vi "medicao.vi"() -> ()   [LabVIEW 2023]
doc: "This example performs writes and reads on a serial port, as directed by the user. You can press the Write and Read buttons, and change the Read Count, while the example is running.\n\nThe parameters set for the serial port must match the parameters of the connected instrument or device. In this example, the Read Count parameter specifies the number of bytes that the serial port reads. If there were more bytes at the port than the specified number, those bytes would not be read. If there were less bytes at the port than the specified number, you would receive a timeout error.\n\nThis example expands upon the flow control options for XON and XOFF, allowing the user to choose those control characters. Also, the user can enable or disable a termination character. Some devices require a termination character in order to identify the end of command strings. Some devices send a termination character to signify the end of data to be read. This example shows how you can end the Read operation once a termination character is detected in the buffer and/or append a termination character at the end of the Write data."
uses:
  <vilib>/Instr/_visa.llb/VISA Flush IO Buffer Mask.ctl
  <vilib>/Instr/_visa.llb/VISA Configure Serial Port (Instr).vi
panel:
  in  "Trigger":dbl step=0.01
  out "Temperatura":cluster{i32, dbl}(graph)
  out "Luminância":cluster{i32, dbl}(graph)
  out "Corrente":cluster{dbl[], dbl[]}(graph)
  out "Potência":cluster{dbl[], dbl[]}(graph)
  out "Tensão":cluster{dbl[], dbl[]}(graph)
  in  "Stop":bool
  in  "VISA resource name":refnum<visa-resource-name>="COM1"
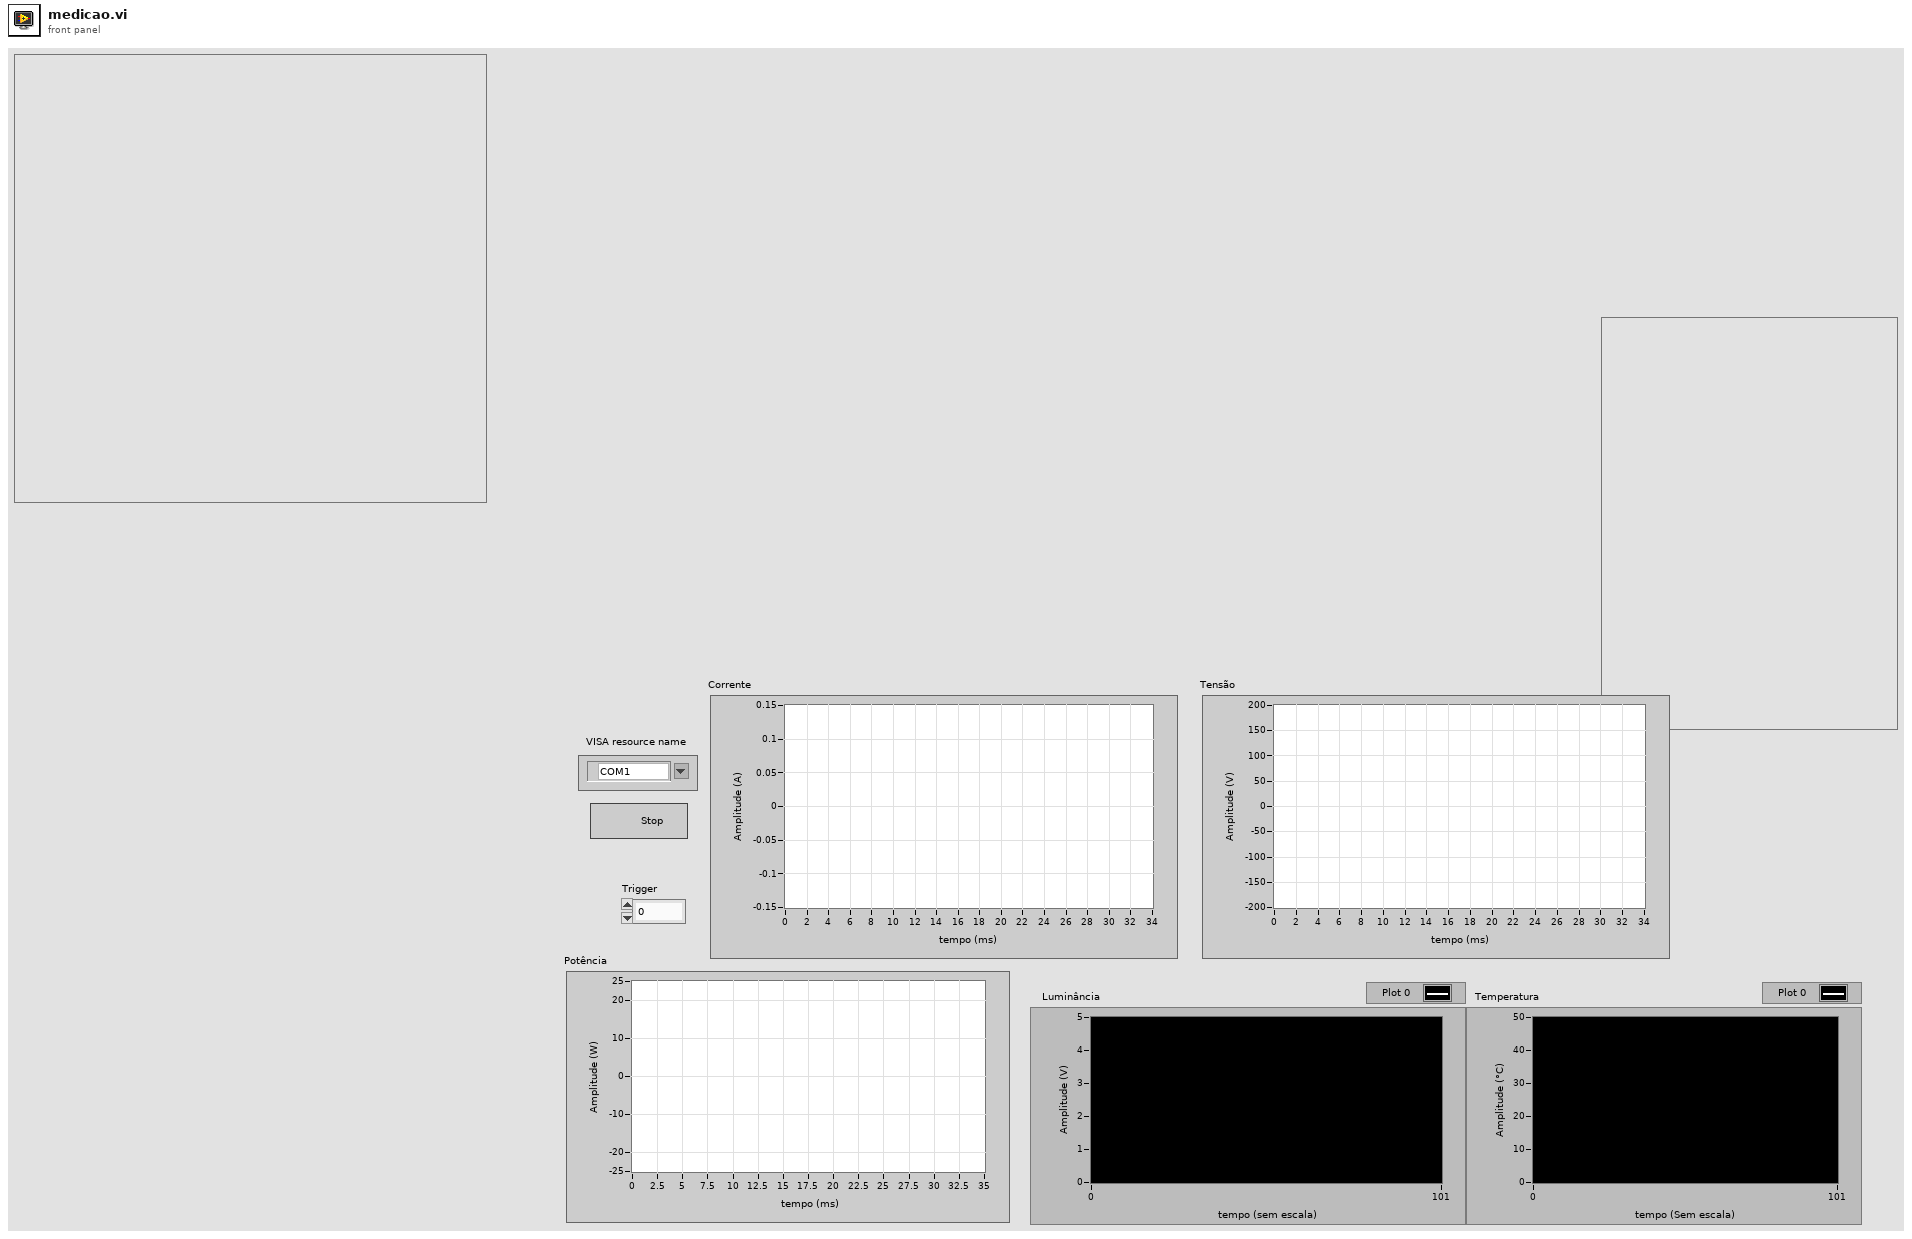
[diagram p1: front panel]
types:
  T1 = typedef "VISA Flush IO Buffer Mask.ctl" = u16
  T2 = cluster{"baud rate":u32, "data bits":u16, "parity":enum16{"None", "Odd", "Even", "Mark", "Space"}, "stop bits":u16, "flow control":u16}
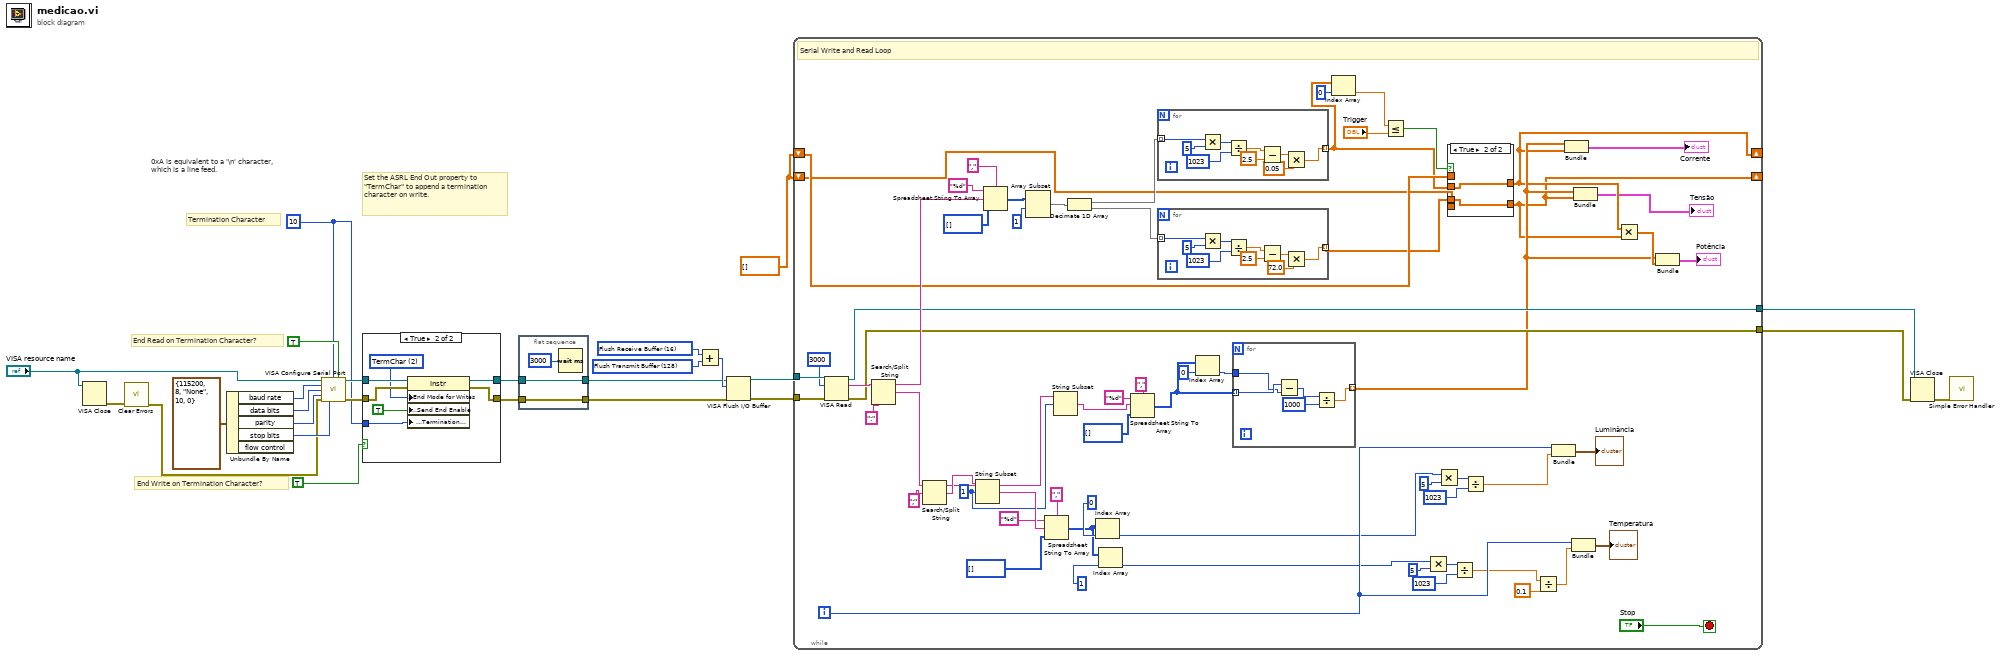
[diagram p0: block diagram]
diagram:
  w1 = dbl[] []
  w17 = T1 128 items=["Flush Receive Buffer"=16, "Write Transmit Buffer to Device"=32, "Flush Receive Buffer (No I/O)"=64, "Flush Transmit Buffer"=128] ("Mask")
  w18 = T1 16 items=["Flush Receive Buffer"=16, "Write Transmit Buffer to Device"=32, "Flush Receive Buffer (No I/O)"=64, "Flush Transmit Buffer"=128] ("Mask")
  w9 = u8 10 ("Termination Character")
  # "0xA is equivalent to a '\\n' character, which is a line feed."
  # "End Write on Termination Character?"
  # "Termination Character"
  # "End Read on Termination Character?"
  # "Set the ASRL End Out property to \"TermChar\" to append a termination character on write."
  n1 = VISA Close(VISA resource name="VISA resource name") -> (error out=w5:errorcluster)  [unwired: 1 in]
  n2 = call <vilib>:"Clear Errors.vi"("error in (no error)"=w5) -> ("error out"=w4:errorcluster)  [unwired: 5 in, 1 out]
  n3 = Unbundle By Name(T2 {"baud rate"=115200, "data bits"=8, "parity"=enum."None", "stop bits"=10, "flow control"=0} ("Serial Settings")) -> ("baud rate"=w23:u32, "data bits"=w24:u16, "parity"=w25:enum16{"None", "Odd", "Even", "Mark", "Space"}, "stop bits"=w26:u16)  [unwired: 1 out]
  n4 = call-poly "VISA Configure Serial Port"("VISA resource name"="VISA resource name", "termination char\n(0xA = '\\n' = LF)"=w9, "Enable Termination\nChar (T)"=TRUE ("End Read on Termination Character?"), "baud rate (9600)"=w23, "data bits (8)"=w24, "parity (0:none)"=w25, "error in (no error)"=w4, "stop bits (10: 1 bit)"=w26) -> ("VISA resource name out"=w11:refnum<visa-resource-name>, "error out"=w10:errorcluster)  [unwired: 2 in, 4 out]
  n5 = case shown="True" TRUE ("End Write on Termination Character?") {
    tunnel: w11 -> [w27 w35]
    tunnel: w10 -> [w28 w34]
    tunnel: [w27 w33] -> w13
    tunnel: [w28 w32] -> w12
    tunnel: w9 -> [_ w30]
    frame False {
    }
    frame True {
      w31 = u16 2 items=["None", "LastBit", "TermChar", "Break"] ("Serial Settings:Serial End Mode for Writes")
      n6 = property class="Instr"(reference=w35, error in=w34, "Serial Settings:End Mode for Writes"=w31, "Message Based Settings:Send End Enable"=TRUE, "Message Based Settings:Termination Character"=w30) -> (reference out=w33:refnum<visa-resource-name>, error out=w32:errorcluster)
    }
  }
  n7 = flat-sequence {
    tunnel: w13 -> [w36]
    tunnel: w12 -> [w37]
    tunnel: [w37] -> w15
    tunnel: [w36] -> w14
    frame #0 {
      n8 = Wait (ms)(milliseconds to wait=u32 3000) -> ()  [unwired: 1 out]
    }
  }
  n9 = Add(x=w18, y=w17) -> (x+y=w16:T1)
  n10 = VISA Flush I/O Buffer(VISA resource name=w14, mask (16)=w16, error in (no error)=w15) -> (VISA resource name out=w8:refnum<visa-resource-name>, error out=w7:errorcluster)
  n11 = while {
    tunnel: w7 -> [w103]
    tunnel: w8 -> [w104]
    tunnel: [w94] -> w3
    tunnel: [w93] -> w2
    shift-right: [w43] -> _
    shift-left: w1 -> [w46]
    shift-right: [w40] -> _
    shift-left: w1 -> [w41]
    i -> [w73]
    stop <- "Stop" stop-if-true
    w79 = 1 ("offset (0)")
    # "Serial Write and Read Loop"
    n12 = VISA Read(VISA resource name=w104, byte count=u32 3000, error in (no error)=w103) -> (VISA resource name out=w94:refnum<visa-resource-name>, read buffer=w102:string, error out=w93:errorcluster)  [unwired: 1 out]
    n13 = Search/Split String(string=w102, search string/char (-)=":") -> (substring before match=w100:string, match + rest of string=w85:string)  [unwired: 1 in, 1 out]
    n14 = Search/Split String(string=w85, search string/char (-)=";") -> (substring before match=w80:string, match + rest of string=w83:string)  [unwired: 1 in, 1 out]
    n15 = String Subset(string=w83, offset (0)=w79) -> (substring=w97:string)  [unwired: 1 in]
    n16 = Spreadsheet String To Array(delimiter (Tab)=",", format string="%d", spreadsheet string=w100, array type (2D Dbl)=u16[] []) -> (array=w86:u16[])
    n17 = Array Subset(array=w86, index=1) -> (w87:u16[])  [unwired: 1 in]
    n18 = Spreadsheet String To Array(delimiter (Tab)=",", format string="%d", spreadsheet string=w97, array type (2D Dbl)=u16[] []) -> (array=w71:u16[])
    n19 = String Subset(string=w80, offset (0)=w79) -> (substring=w78:string)  [unwired: 1 in]
    n20 = Decimate 1D Array(w87) -> (w68:u16[], w65:u16[])
    n21 = Index Array(array=w71, index=0) -> (element=w53:u16)
    n22 = Index Array(array=w71, index=1) -> (element=w61:u16)
    n23 = Spreadsheet String To Array(delimiter (Tab)=",", format string="%d", spreadsheet string=w78, array type (2D Dbl)=u32[] []) -> (array=w75:u32[])
    n24 = for {
      tunnel: w68 -> [w117] mode=indexing
      tunnel: [w109] -> w45 mode=indexing
      n25 = Multiply(x=w117, y=u16 5) -> (x*y=w115:u16)
      n26 = Divide(x=w115, y=u16 1023) -> (x/y=w113:dbl)
      n27 = Subtract(x=w113, y=2.5) -> (x-y=w111:dbl)
      n28 = Multiply(x=w111, y=0.05) -> (x*y=w109:dbl)
    }
    n29 = for {
      tunnel: w65 -> [w126] mode=indexing
      tunnel: [w118] -> w42 mode=indexing
      n30 = Multiply(x=w126, y=u16 5) -> (x*y=w124:u16)
      n31 = Divide(x=w124, y=u16 1023) -> (x/y=w122:dbl)
      n32 = Subtract(x=w122, y=2.5) -> (x-y=w120:dbl)
      n33 = Multiply(x=w120, y=72.0) -> (x*y=w118:dbl)
    }
    n34 = Index Array(array=w75, index=0) -> (element=w74:u32)
    n35 = for {
      tunnel: w75 -> [w131] mode=indexing
      tunnel: w74 -> [w130]
      tunnel: [w128] -> w51 mode=indexing
      n36 = Subtract(x=w131, y=w130) -> (x-y=w129:u32)
      n37 = Divide(x=w129, y=u32 1000) -> (x/y=w128:dbl)
    }
    n38 = Index Array(array=w45, index=0) -> (element=w49:dbl)
    n39 = Less Or Equal?(x=w49, y="Trigger") -> (x <= y?=w44:bool)
    n40 = Multiply(x=w61, y=u16 5) -> (x*y=w63:u16)
    n41 = Multiply(x=w53, y=u16 5) -> (x*y=w55:u16)
    n42 = case shown="True" w44 {
      tunnel: w46 -> [w106 _]
      tunnel: w45 -> [_ w108]
      tunnel: [w106 w108] -> w43
      tunnel: w42 -> [_ w107]
      tunnel: w41 -> [w105 _]
      tunnel: [w105 w107] -> w40
      frame False {
      }
      frame True {
      }
    }
    n43 = Divide(x=w63, y=u16 1023) -> (x/y=w58:dbl)
    n44 = Divide(x=w55, y=u16 1023) -> (x/y=w52:dbl)
    n45 = Divide(x=w58, y=0.1) -> (x/y=w57:dbl)
    n46 = Bundle(w73, w52) -> (→"Luminância":cluster{i32, dbl})  [unwired: 1 in]
    n47 = Bundle(w51, w43) -> (→"Corrente":cluster{dbl[], dbl[]})  [unwired: 1 in]
    n48 = Bundle(w73, w57) -> (→"Temperatura":cluster{i32, dbl})  [unwired: 1 in]
    n49 = Bundle(w51, w40) -> (→"Tensão":cluster{dbl[], dbl[]})  [unwired: 1 in]
    n50 = Multiply(x=w43, y=w40) -> (x*y=w67:dbl[])
    n51 = Bundle(w51, w67) -> (→"Potência":cluster{dbl[], dbl[]})  [unwired: 1 in]
  }
  n52 = VISA Close(VISA resource name=w3, error in (no error)=w2) -> (error out=w19:errorcluster)
  n53 = call <vilib>:"Simple Error Handler.vi"("error in (no error)"=w19) -> ()  [unwired: 1 in, 8 out]
